vi "NP_Control.vi"(8 "error in (no error)":errorcluster, 9 "Color Box":u32(colorbox), 11 "VISA resource name":refnum<visa-resource-name>) -> (0 "error out":errorcluster, 3 "VISA resource name out":refnum<visa-resource-name>)   [LabVIEW 2025]
doc: "VI que permite utilizar las 3 Neo Pixel y asignarles un mismo color \nSe puede enviar el numero de 32 bits o usar la color box\nNo requiere input de pin ya que asume que se esta utilizando la placa Galiot de universidad Galileo"
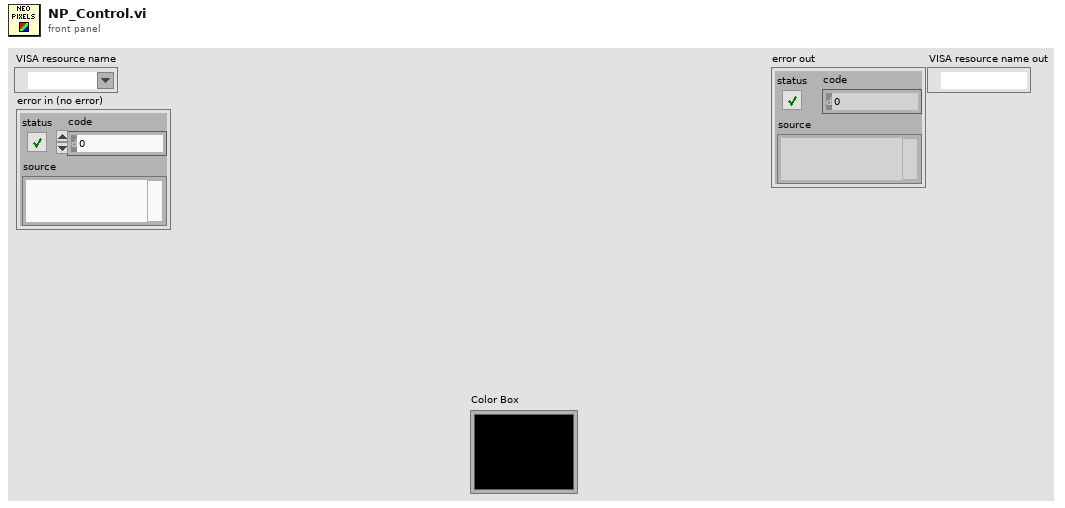
[diagram p1: front panel]
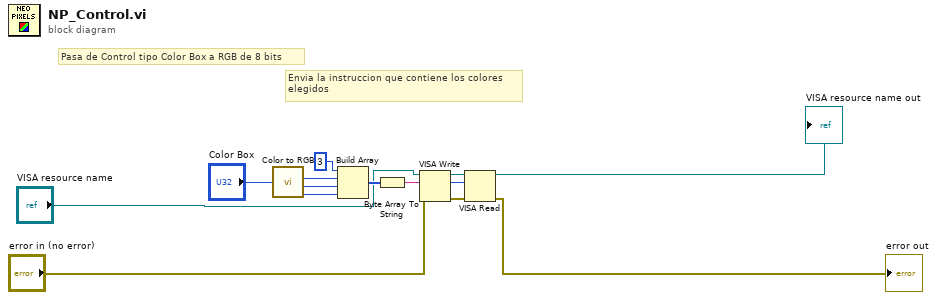
[diagram p0: block diagram]
diagram:
  # "Envia la instruccion que contiene los colores\nelegidos"
  # "Pasa de Control tipo Color Box a RGB de 8 bits"
  n1 = call <vilib>:"Color to RGB.vi"("Color"="Color Box") -> ("R"=w10:u8, "G"=w9:u8, "B"=w8:u8)  [unwired: 1 out]
  n2 = Build Array(u8 3 ("element"), w10, w9, w8) -> (w6:u8[])
  n3 = Byte Array To String(unsigned byte array=w6) -> (string=w14:string)
  n4 = VISA Write(VISA resource name="VISA resource name", write buffer=w14, error in (no error)="error in (no error)") -> (VISA resource name out=w12:refnum<visa-resource-name>, return count=w5:u32, error out=w13:errorcluster)
  n5 = VISA Read(VISA resource name=w12, byte count=w5, error in (no error)=w13) -> (VISA resource name out=→"VISA resource name out":refnum<visa-resource-name>, error out=→"error out":errorcluster)  [unwired: 2 out]
